vi "HumanTrajPositionsDash.vi"(11 "Init":bool) -> (1 "vAngular":dbl, 2 "vY":dbl, 3 "vX":dbl)   [LabVIEW 2023]
uses:
  <vilib>/Rock Robotics/WPI/ThirdParty/JAS_Junk/TrajLib/Trajectory_Library.lvlib
  HumanGlobal.vi
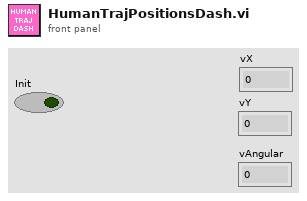
[diagram p1: front panel]
types:
  T1 = typedef "Trajectory_Library.lvlib/POSE2D.ctl" = cluster{"TRANSLATION":T2, "ROTATION":T3}
  T2 = typedef "Trajectory_Library.lvlib/TRANSLATION2D.ctl" = cluster{"X":dbl, "Y":dbl}
  T3 = typedef "Trajectory_Library.lvlib/ROTATION2D.ctl" = cluster{"VALUE":dbl, "COS":dbl, "SIN":dbl}
  T4 = typedef "Trajectory_Library.lvlib/CHASSIS_SPEEDS.ctl" = cluster{"vX":dbl, "vY":dbl, "vOmega":dbl}
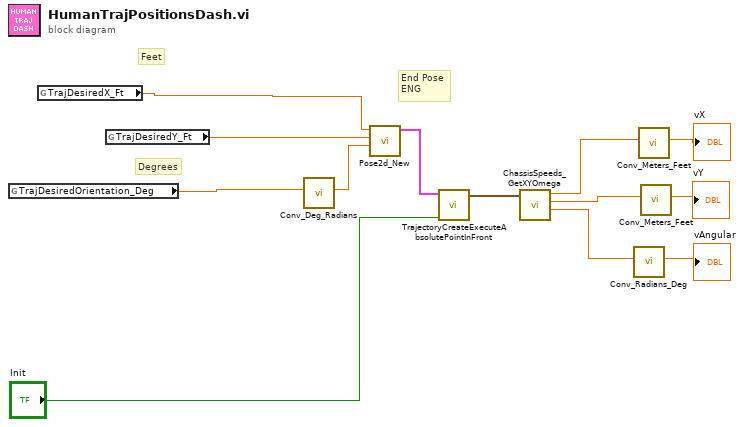
[diagram p0: block diagram]
diagram:
  # "End Pose\nENG"
  # "Degrees"
  # "Feet"
  n1 = global read "HumanGlobal.vi" "TrajDesiredOrientation_Deg"() -> (w1:dbl)
  n2 = global read "HumanGlobal.vi" "TrajDesiredX_Ft"() -> (w3:dbl)
  n3 = global read "HumanGlobal.vi" "TrajDesiredY_Ft"() -> (w2:dbl)
  n4 = call <vilib>:"Conv_Deg_Radians.vi"("Degress"=w1) -> ("Radians"=w4:dbl)  [unwired: 10 in]
  n5 = call <vilib>:"Pose2d_New.vi"("Heading"=w4, "Y"=w2, "X"=w3) -> ("out POSe"=w13:T1)  [unwired: 8 in]
  n6 = call "TrajectoryCreateExecuteAbsolutePointInFront.vi"("Init"="Init", "End Pose ENG"=w13) -> ("Chassis Velocity Target"=w12:T4)  [unwired: 8 in, 1 out]
  n7 = call <vilib>:"ChassisSpeeds_GetXYOmega.vi"("CHASSIS"=w12) -> ("vAngular"=w5:dbl, "vY"=w9:dbl, "vX"=w10:dbl)  [unwired: 8 in]
  n8 = call <vilib>:"Conv_Radians_Deg.vi"("Radians"=w5) -> ("Degrees"=→"vAngular":dbl)  [unwired: 10 in]
  n9 = call <vilib>:"Conv_Meters_Feet.vi"("Meters"=w10) -> ("Feet"=→"vX":dbl)  [unwired: 10 in]
  n10 = call <vilib>:"Conv_Meters_Feet.vi"("Meters"=w9) -> ("Feet"=→"vY":dbl)  [unwired: 10 in]
